vi "fpga_feedback_error.vi"(7 "feedback config":T2, 11 "AI":T1) -> (0 "process variable":sgl, 2 "ready to move?":bool, 3 "feedback error":sgl)   [LabVIEW 2021]
doc: "Calculate the feedback error with setpoint and actual input."
uses:
  fpga_feedback_config.ctl
  fpga_dtype_sgl_8ch.ctl
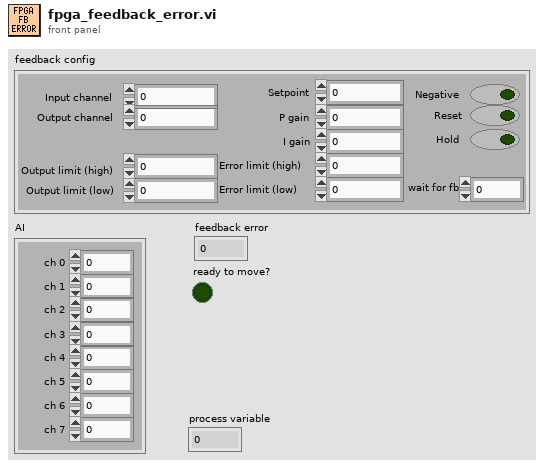
[diagram p1: front panel]
types:
  T1 = typedef "fpga_dtype_sgl_8ch.ctl" = cluster{"ch 0":sgl, "ch 1":sgl, "ch 2":sgl, "ch 3":sgl, "ch 4":sgl, "ch 5":sgl, "ch 6":sgl, "ch 7":sgl}
  T2 = typedef "fpga_feedback_config.ctl" = cluster{"Setpoint":sgl, "Output limit (low)":sgl, "Output limit (high)":sgl, "P gain":sgl, "I gain":sgl, "Reset":bool, "Hold":bool, "Negative":bool, "Input channel":i16, "Output channel":i16, "wait for fb":i16, "Error limit (high)":sgl, "Error limit (low)":sgl}
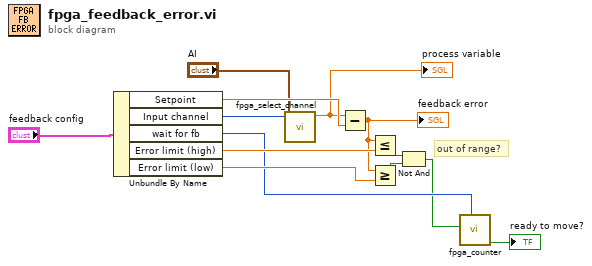
[diagram p0: block diagram]
diagram:
  # "out of range?"
  n1 = Unbundle By Name("feedback config") -> ("Setpoint"=w12:sgl, "Input channel"=w13:i16, "wait for fb"=w3:i16, "Error limit (high)"=w9:sgl, "Error limit (low)"=w8:sgl)
  n2 = call "fpga_select_channel.vi"("sgl 8ch"="AI", "channel"=w13) -> ("value"=w4:sgl)  [unwired: 9 in]
  "process variable" <- w4
  n3 = Subtract(x=w4, y=w12) -> (x-y=w5:sgl)
  "feedback error" <- w5
  n4 = Less Or Equal?(x=w5, y=w9) -> (x <= y?=w11:bool)
  n5 = Greater Or Equal?(x=w5, y=w8) -> (x >= y?=w10:bool)
  n6 = Not And(1:w10, 2:w11) -> (0:w2:bool)
  n7 = call "fpga_counter.vi"("max counts"=w3, "reset? (F)"=w2) -> ("completed? (switch)"=→"ready to move?":bool)  [unwired: 8 in, 1 out]
